vi "Write Measurement Settings.vi"(8 "error in":errorcluster, 10 "Measurement Settings":T1, 11 "Instrument Driver in":refnum<class "Instrument Driver.lvclass">) -> (0 "error out":errorcluster, 3 "Instrument Driver out":refnum<class "Instrument Driver.lvclass">)   [LabVIEW 2020, in "Plugin Instrument Driver.lvlib" / "Instrument Driver.lvclass"]
doc: "Write Measurement Settings"
uses:
  Instrument Driver.lvclass
  Typedefs/Measurement Settings.ctl
  Instrument Driver.lvclass/Instrument Driver.ctl
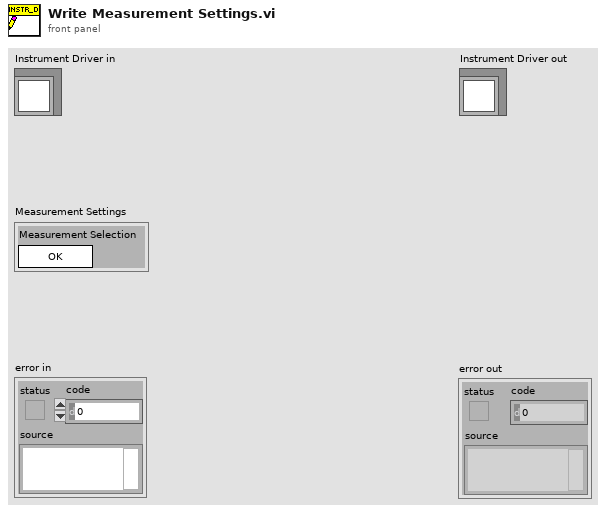
[diagram p1: front panel]
types:
  T1 = typedef "Plugin Instrument Driver.lvlib/Instrument Driver.lvclass/Measurement Settings.ctl" = cluster{"Measurement Selection":bool}
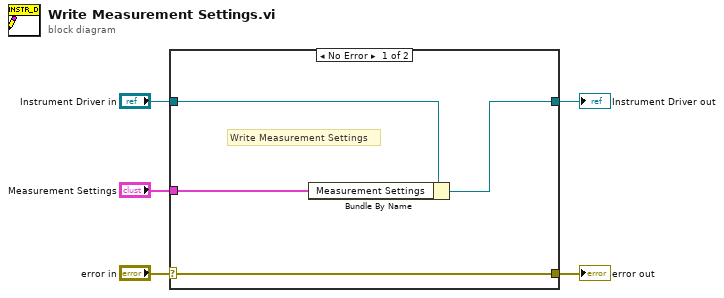
[diagram p0: block diagram]
diagram:
  n1 = case shown="No Error" "error in" {
    selector: "error in" -> [w9 w10]
    tunnel: [w9 w10] -> w4
    tunnel: [w7 w11] -> w2
    tunnel: "Instrument Driver in" -> [w8 w11]
    tunnel: "Measurement Settings" -> [w6 _]
    frame No Error {
      # "Write Measurement Settings"
      n2 = Bundle By Name(cluster=w8, "Measurement Settings"=w6) -> (w7:refnum<class "Instrument Driver.lvclass">)
    }
    frame Error {
    }
  }
  "error out" <- w4
  "Instrument Driver out" <- w2
